vi "process.vi"(8 "error in":errorcluster, 9 "result allocation":T1, 10 "parameters":T1, 11 "module in":refnum<class "Increment runtime.lvclass">) -> (0 "error out":errorcluster, 1 "results":T1, 2 "parameter allocation":T1, 3 "module out":refnum<class "Increment runtime.lvclass">)   [LabVIEW 2015, in "Increment runtime.lvclass"]
doc: "Provides an interface for information processing by a module at runtime. While this interface performs no operations, a child should provide an override which may process data in any manner necessary."
uses:
  Increment runtime.lvclass
  <vilib>/NI/Tag Bus/table/data table.ctl
  Increment runtime.lvclass/Increment runtime.ctl
  <vilib>/NI/Tag Bus/table/data polymorphs/read one/read Double.vi
  <vilib>/NI/Tag Bus/table/data polymorphs/write one/write Double.vi
  <vilib>/NI/Tag Bus/table/data table.lvlib
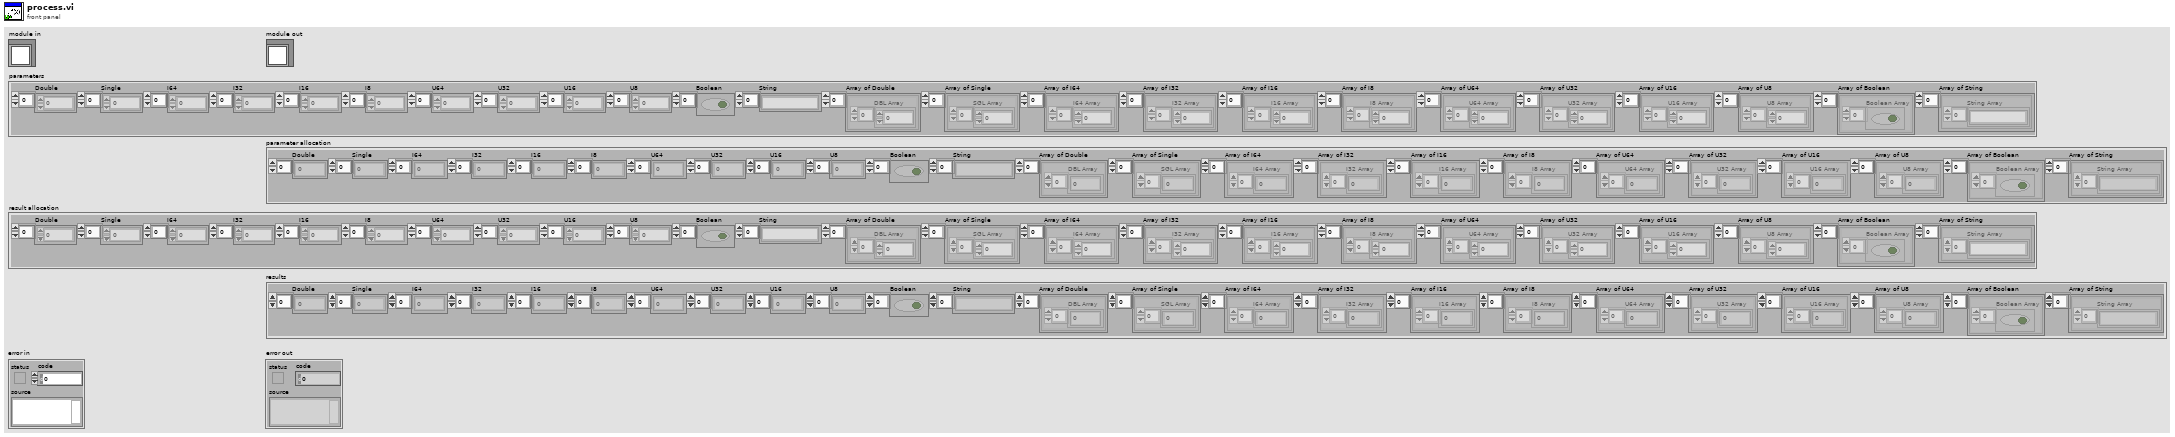
[diagram p1: front panel]
types:
  T1 = typedef "tag bus.lvlib/data table.lvlib/data table.ctl" = cluster{"Double":dbl[], "Single":sgl[], "I64":i64[], "I32":i32[], "I16":i16[], "I8":i8[], "U64":u64[], "U32":u32[], "U16":u16[], "U8":u8[], "Boolean":bool[], "String":string[], "Array of Double":cluster{"DBL Array":dbl[]}[], "Array of Single":cluster{"SGL Array":sgl[]}[], "Array of I64":cluster{"I64 Array":i64[]}[], "Array of I32":cluster{"I32 Array":i32[]}[], "Array of I16":cluster{"I16 Array":i16[]}[], "Array of I8":cluster{"I8 Array":i8[]}[], "Array of U64":cluster{"U64 Array":u64[]}[], "Array of U32":cluster{"U32 Array":u32[]}[], "Array of U16":cluster{"U16 Array":u16[]}[], "Array of U8":cluster{"U8 Array":u8[]}[], "Array of Boolean":cluster{"Boolean Array":bool[]}[], "Array of String":cluster{"String Array":string[]}[]}
  T2 = typedef "Increment runtime.lvclass/Runtime_Mapping.ctl" = cluster{"In Index":i32, "Out Index":i32}
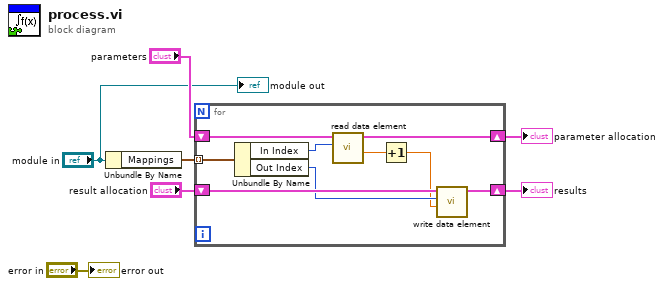
[diagram p0: block diagram]
diagram:
  n1 = Unbundle By Name("module in") -> ("Mappings"=w7:T2[])
  n2 = for {
    tunnel: w7 -> [w12] mode=indexing
    shift-right: [w15] -> w5
    shift-left: "result allocation" -> [w16]
    shift-right: [w13] -> w3
    shift-left: "parameters" -> [w14]
    n3 = Unbundle By Name(w12) -> ("In Index"=w11:i32, "Out Index"=w10:i32)
    n4 = call-poly <vilib>:"read data element.vi"("index"=w11, "data table in"=w14) -> ("value"=w9:dbl, "data table out"=w13:T1)  [unwired: 8 in]
    n5 = Increment(x=w9) -> (x+1=w8:dbl)
    n6 = call-poly <vilib>:"write data element.vi"("value"=w8, "index"=w10, "data table in"=w16) -> ("data table out"=w15:T1)  [unwired: 8 in]
  }
  "results" <- w5
  "parameter allocation" <- w3
  "error out" <- "error in"
  "module out" <- "module in"
